vi "PH_Beamline_Chief.set i Attr and create DIM Services.vi"(0 "Refnum in":refnum<vi>, 5 "error in":errorcluster) -> (14 "i ref out":refnum<vi>, 17 "i Attr":T1={"BL Service IDs"={"YLF_BL_Status"=-1, "fs_BL_Status"=-1, "fs_YLF_BL_Status"=-1, "ns_BL_Status"=-1, "PA_Input_BL_Status"=-1, "PA_UnDelay_BL_Status"=-1, "PA_Delay_BL_Status"=-1, "PA_BL_Status"=-1, "PA_Bypass_BL_Status"=-1, "PA_Exit_BL_Status"=-1, "PA_LL_BL_Status"=-1, "LL_BL_Status"=-1, "PA_MA_BL_Status"=-1, "MA_Exit_BL_Status"=-1, "MA_Z6_BL_Status"=-1, "Z6_BL_Status"=-1, "MA_LB_BL_Status"=-1, "LB_TB2_BL_Status"=-1, "PA_before_Bypass_BL_Status"=-1, "LB_TB3_BL_Status"=-1}, "R2S Service ID"=-1, "Settings"={"Wanted"={"PA Doublepass Mode"=FALSE, "Compressor Vaccuum LB not relevant"=FALSE, "Windowshutter TB2 not relevant"=FALSE, "Windowshutter TB3 not relevant"=FALSE}, "GUI Ref"=refnum, "Service ID"=-1}}, 19 "error out":errorcluster)   [LabVIEW 2014, in "PH_Beamline_Chief.lvlib"]
doc: "This VI creates DIM services."
uses:
  PH_Beamline_Chief.lvlib
  PH_Beamline_Chief.i attribute.ctl
  PH_Beamline_Chief.Settings.ctl
  PH_Beamline_Chief.Section.ctl
  PH_Basics/PH_Common/PH_Common.lvlib
  CSlibraries-extern/DimLVEvent/LVDimInterface/LVDimInterface.lvlib
  CS_Core/CSSystem/CSSystemLib/CSSystemLib.lvlib
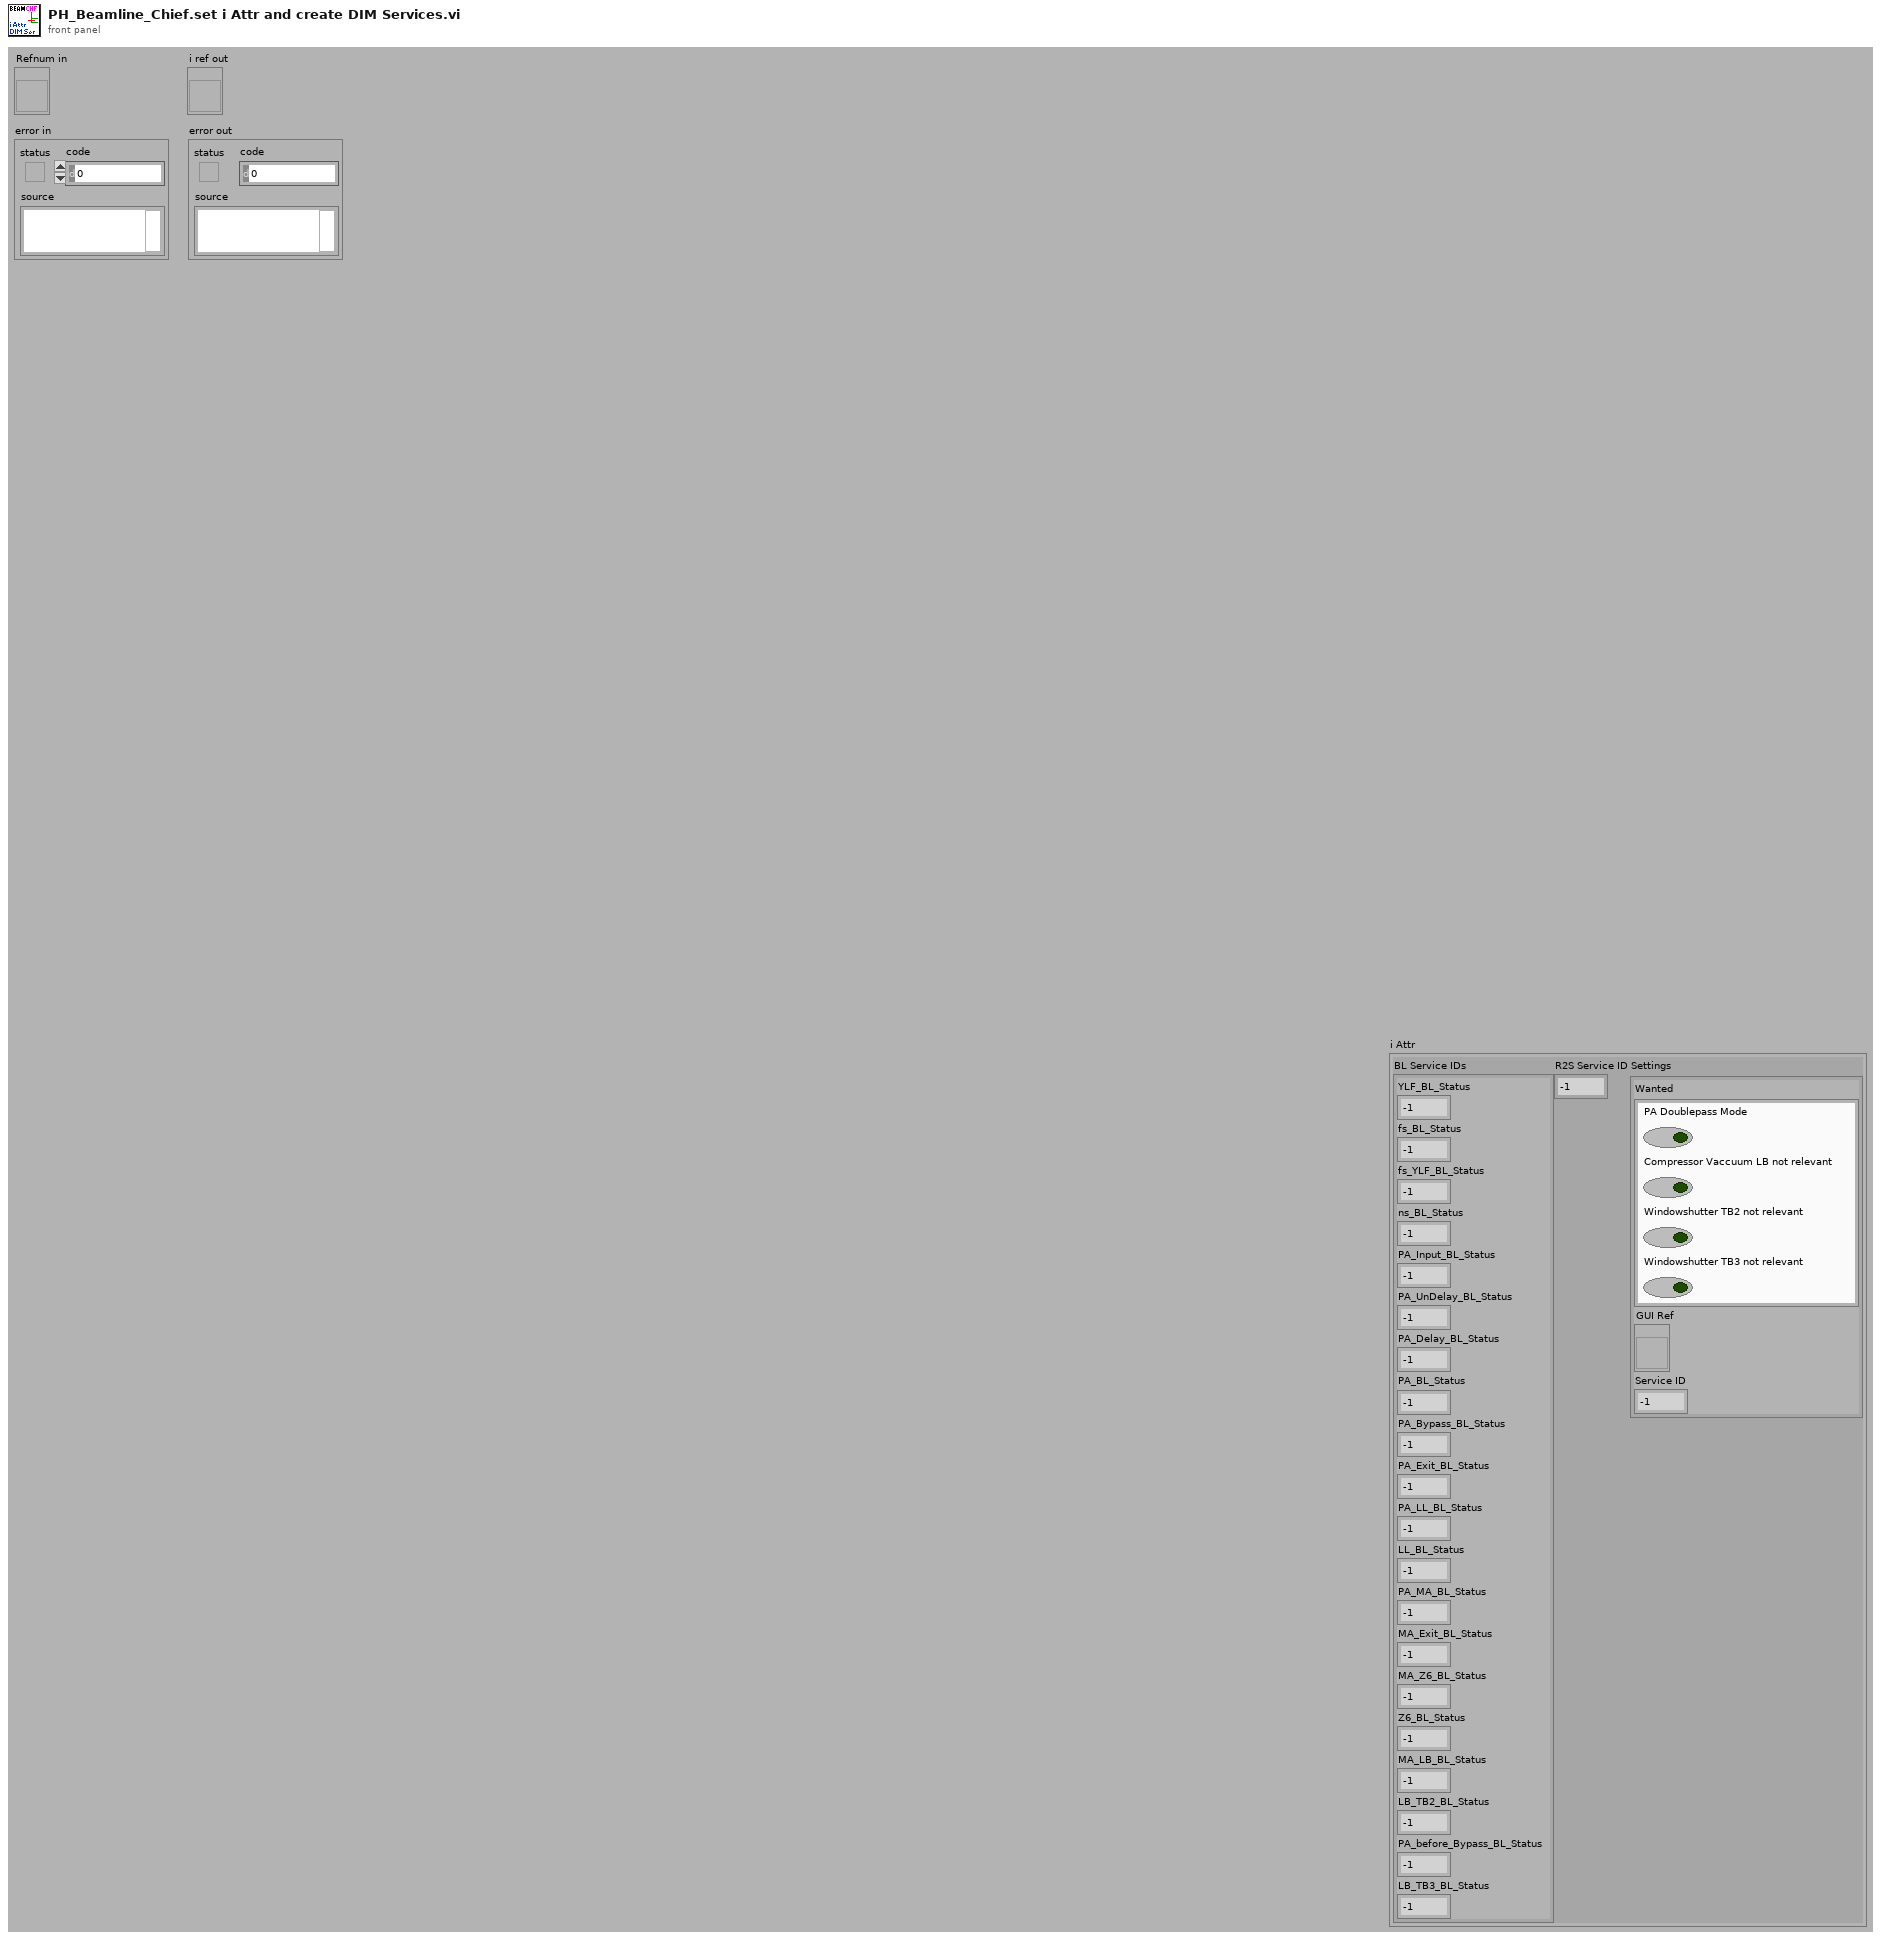
[diagram p1: front panel]
types:
  T1 = typedef "PH_Beamline_Chief.lvlib/PH_Beamline_Chief.i attribute.ctl" = cluster{"BL Service IDs":cluster{"YLF_BL_Status":i32, "fs_BL_Status":i32, "fs_YLF_BL_Status":i32, "ns_BL_Status":i32, "PA_Input_BL_Status":i32, "PA_UnDelay_BL_Status":i32, "PA_Delay_BL_Status":i32, "PA_BL_Status":i32, "PA_Bypass_BL_Status":i32, "PA_Exit_BL_Status":i32, "PA_LL_BL_Status":i32, "LL_BL_Status":i32, "PA_MA_BL_Status":i32, "MA_Exit_BL_Status":i32, "MA_Z6_BL_Status":i32, "Z6_BL_Status":i32, "MA_LB_BL_Status":i32, "LB_TB2_BL_Status":i32, "PA_before_Bypass_BL_Status":i32, "LB_TB3_BL_Status":i32}, "R2S Service ID":i32, "Settings":cluster{"Wanted":T2, "GUI Ref":refnum<vi>, "Service ID":i32}}
  T2 = typedef "PH_Beamline_Chief.lvlib/PH_Beamline_Chief.Settings.ctl" = cluster{"PA Doublepass Mode":bool, "Compressor Vaccuum LB not relevant":bool, "Windowshutter TB2 not relevant":bool, "Windowshutter TB3 not relevant":bool}
  T3 = typedef "PH_Beamline_Chief.lvlib/PH_Beamline_Chief.Section.ctl" = enum16{"None", "YLF", "fs", "fs-YLF", "ns", "PA-Input", "PA-Undelay", "PA-Delay", "PA-before-Bypass", "PA", "PA-Bypass", "PA-Exit", "PA-LL", "LL", "PA-MA", "MA-Exit", "MA-Z6", "Z6", "MA-LB", "LB-TB2", "LB-TB3"}
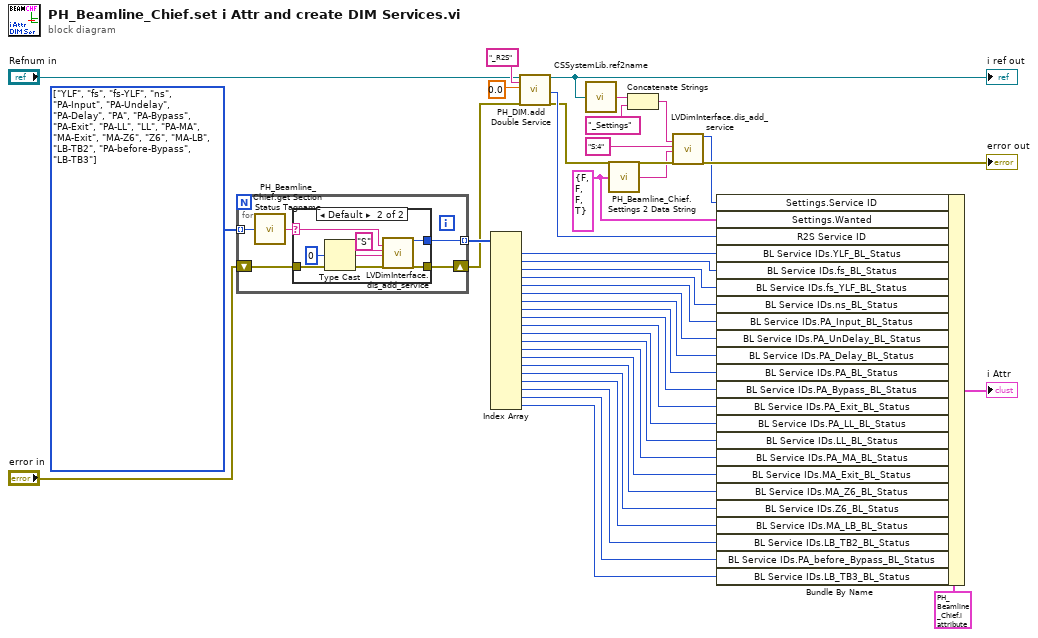
[diagram p0: block diagram]
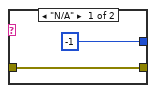
[diagram p2: hidden frame]
diagram:
  w3 = T2 {"PA Doublepass Mode"=FALSE, "Compressor Vaccuum LB not relevant"=FALSE, "Windowshutter TB2 not relevant"=FALSE, "Windowshutter TB3 not relevant"=TRUE} ("Settings.Wanted")
  w17 = T3[] [enum."YLF", enum."fs", enum."fs-YLF", enum."ns", enum."PA-Input", enum."PA-Undelay", enum."PA-Delay", enum."PA", enum."PA-Bypass", enum."PA-Exit", enum."PA-LL", enum."LL", enum."PA-MA", enum."MA-Exit", enum."MA-Z6", enum."Z6", enum."MA-LB", enum."LB-TB2", enum."PA-before-Bypass", enum."LB-TB3"] items=["None", "YLF", "fs", "fs-YLF", "ns", "PA-Input", "PA-Undelay", "PA-Delay", "PA-before-Bypass", "PA", "PA-Bypass", "PA-Exit", "PA-LL", "LL", "PA-MA", "MA-Exit", "MA-Z6", "Z6", "MA-LB", "LB-TB2", "LB-TB3"]
  n1 = for {
    tunnel: w17 -> [w45] mode=indexing
    shift-right: [w41] -> w13
    shift-left: "error in" -> [w42]
    tunnel: [w43] -> w16 mode=indexing
    n2 = call "PH_Beamline_Chief.get Section Status Tagname.vi"("Beamline Section"=w45) -> ("Section Status Tagname"=w44:string)
    n3 = case shown="Default" w44 {
      selector: w44 -> [_ w49]
      tunnel: [-1 ("my_serviceID") w50] -> w43
      tunnel: [w47 w51] -> w41
      tunnel: w42 -> [w47 w52]
      frame "N/A" {
      }
      frame Default {
        n4 = Type Cast(x=i16 0 ("Number")) -> (*(type *) &x=w54:string)  [unwired: 1 in]
        n5 = call "LVDimInterface.dis_add_service.vi"("serviceName"=w49, "typeDescriptor"="S", "data"=w54, "error in (no error)"=w52) -> ("my_serviceID"=w50:i32, "error out"=w51:errorcluster)  [unwired: 14 in]
      }
    }
  }
  n6 = Index Array(array=w16) -> (element #1=w23:i32, element #2=w24:i32, element #3=w25:i32, element #4=w26:i32, element #5=w27:i32, element #6=w28:i32, element #7=w29:i32, element #8=w30:i32, element #9=w31:i32, element #10=w32:i32, element #11=w33:i32, element #12=w34:i32, element #13=w35:i32, element #14=w36:i32, element #15=w37:i32, element #16=w38:i32, element #17=w39:i32, element #18=w40:i32, element #19=w21:i32, element #20=w20:i32)  [unwired: 20 in]
  n7 = call "PH_DIM.add Double Service.vi"("i ref in"="Refnum in", "Service Name"="_R2S" ("string"), "Double Value"=0.0 ("x"), "error in (no error)"=w13) -> ("i ref out"=w6:refnum<vi>, "Service ID"=w12:i32, "error out"=w11:errorcluster)  [unwired: 13 in]
  "i ref out" <- w6
  n8 = call "CSSystemLib.ref2name.vi"("obj refnum"=w6) -> ("name"=w7:string)
  n9 = call "PH_Beamline_Chief.Settings 2 Data String.vi"("Settings"=w3) -> ("Data String"=w2:string)
  n10 = Concatenate Strings(w7, "_Settings" ("string")) -> (w4:string)
  n11 = call "LVDimInterface.dis_add_service.vi"("serviceName"=w4, "typeDescriptor"="S:4", "data"=w2, "error in (no error)"=w11) -> ("my_serviceID"=w9:i32, "error out"=→"error out":errorcluster)  [unwired: 14 in]
  n12 = Bundle By Name(cluster=T1 {"BL Service IDs"={"YLF_BL_Status"=-1, "fs_BL_Status"=-1, "fs_YLF_BL_Status"=-1, "ns_BL_Status"=-1, "PA_Input_BL_Status"=-1, "PA_UnDelay_BL_Status"=-1, "PA_Delay_BL_Status"=-1, "PA_BL_Status"=-1, "PA_Bypass_BL_Status"=-1, "PA_Exit_BL_Status"=-1, "PA_LL_BL_Status"=-1, "LL_BL_Status"=-1, "PA_MA_BL_Status"=-1, "MA_Exit_BL_Status"=-1, "MA_Z6_BL_Status"=-1, "Z6_BL_Status"=-1, "MA_LB_BL_Status"=-1, "LB_TB2_BL_Status"=-1, "PA_before_Bypass_BL_Status"=-1, "LB_TB3_BL_Status"=-1}, "R2S Service ID"=-1, "Settings"={"Wanted"={"PA Doublepass Mode"=FALSE, "Compressor Vaccuum LB not relevant"=FALSE, "Windowshutter TB2 not relevant"=FALSE, "Windowshutter TB3 not relevant"=FALSE}, "GUI Ref"=refnum, "Service ID"=-1}} ("i attribute"), "Settings.Service ID"=w9, "Settings.Wanted"=w3, "R2S Service ID"=w12, "BL Service IDs.YLF_BL_Status"=w23, "BL Service IDs.fs_BL_Status"=w24, "BL Service IDs.fs_YLF_BL_Status"=w25, "BL Service IDs.ns_BL_Status"=w26, "BL Service IDs.PA_Input_BL_Status"=w27, "BL Service IDs.PA_UnDelay_BL_Status"=w28, "BL Service IDs.PA_Delay_BL_Status"=w29, "BL Service IDs.PA_BL_Status"=w30, "BL Service IDs.PA_Bypass_BL_Status"=w31, "BL Service IDs.PA_Exit_BL_Status"=w32, "BL Service IDs.PA_LL_BL_Status"=w33, "BL Service IDs.LL_BL_Status"=w34, "BL Service IDs.PA_MA_BL_Status"=w35, "BL Service IDs.MA_Exit_BL_Status"=w36, "BL Service IDs.MA_Z6_BL_Status"=w37, "BL Service IDs.Z6_BL_Status"=w38, "BL Service IDs.MA_LB_BL_Status"=w39, "BL Service IDs.LB_TB2_BL_Status"=w40, "BL Service IDs.PA_before_Bypass_BL_Status"=w21, "BL Service IDs.LB_TB3_BL_Status"=w20) -> (→"i Attr":T1)
